vi "两边沿间隔_单点.vi"() -> ()   [LabVIEW 2013]
uses:
  <userlib>/ArtDAQ/_SubVI/ArtDAQ_CreateCITwoEdgeSepChan.vi
  <userlib>/ArtDAQ/_SubVI/ArtDAQ_Read Counter DBL 1Samp.vi
panel:
  out "H":dbl
  in  "第二个边沿":i32(ring)=10280 items=["上升"=10280, "下降"=10171]
  in  "第一个边沿":i32(ring)=10280 items=["上升"=10280, "下降"=10171]
  in  "Stop":bool
  in  "计数器":string="Dev1/ctr0"
  in  "最小值":dbl=1e-06 format="%0.6f"
  in  "MaxValue":dbl=10.0 caption="最大值" format="%0.6f"
  out "错误输出":errorcluster
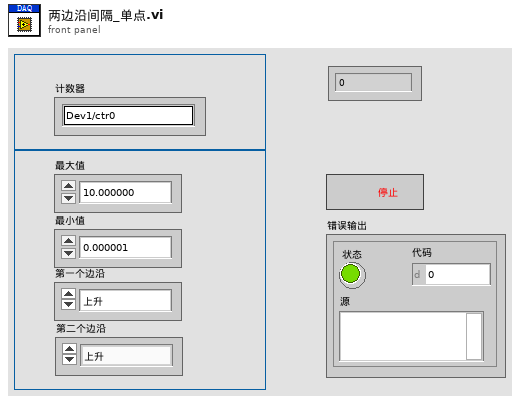
[diagram p1: front panel]
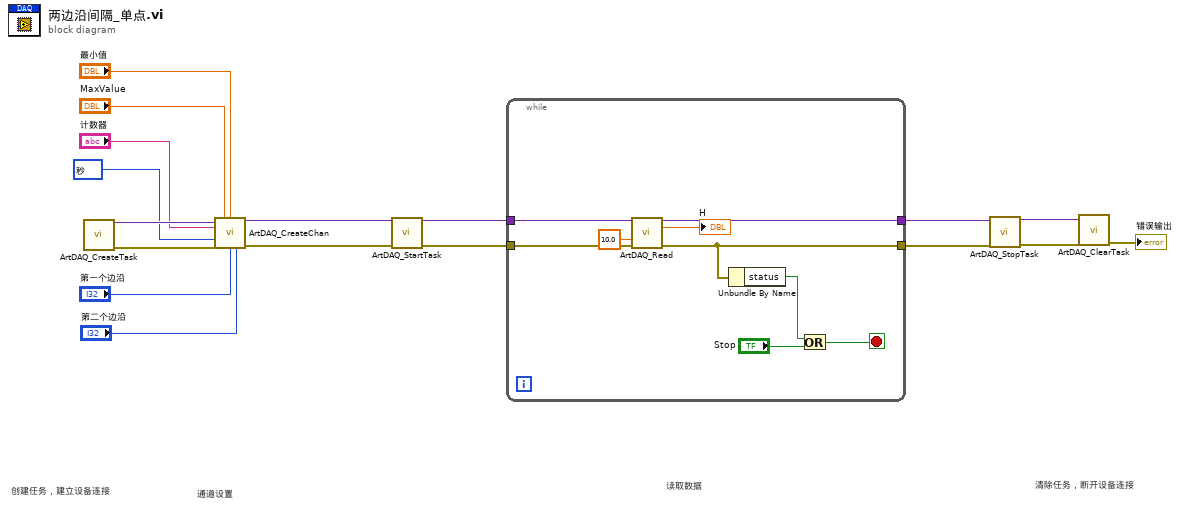
[diagram p0: block diagram]
diagram:
  w7 = 10364 items=["秒"=10364, "时钟滴答"=10304, "来自自定义换算"=10065] ("Units")
  # "清除任务，断开设备连接"
  # "读取数据"
  # "通道设置"
  # "创建任务，建立设备连接"
  n1 = call <userlib>:"ArtDAQ_CreateTask.vi"() -> ("任务句柄"=w17:variant, "错误输出"=w16:errorcluster)  [unwired: 14 in]
  n2 = call-poly <userlib>:"ArtDAQ_CreateChan.vi"("任务句柄"=w17, "最大值"="MaxValue", "最小值"="最小值", "计数器"="计数器", "单位"=w7, "错误输入"=w16, "第一个边沿"="第一个边沿", "第二个边沿"="第二个边沿") -> ("任务句柄"=w2:variant, "错误输出"=w1:errorcluster)  [unwired: 6 in]
  n3 = call <userlib>:"ArtDAQ_StartTask.vi"("任务句柄"=w2, "错误输入"=w1) -> ("任务句柄"=w4:variant, "错误输出"=w3:errorcluster)  [unwired: 12 in]
  n4 = while {
    tunnel: [w26] -> w14
    tunnel: [w25] -> w12
    tunnel: w4 -> [w24]
    tunnel: w3 -> [w23]
    stop <- w19 stop-if-true
    n5 = call-poly <userlib>:"ArtDAQ_Read.vi"("任务句柄"=w24, "超时s"=10.0 ("Timeout"), "错误输入"=w23) -> ("任务句柄"=w26:variant, "数据"=→"H":dbl, "错误输出"=w25:errorcluster)  [unwired: 10 in]
    n6 = Unbundle By Name(w25) -> ("status"=w21:bool)
    n7 = Or(x=w21, y="Stop") -> (x .or. y?=w19:bool)
  }
  n8 = call <userlib>:"ArtDAQ_StopTask.vi"("任务句柄"=w14, "错误输入"=w12) -> ("任务句柄"=w13:variant, "错误输出"=w11:errorcluster)  [unwired: 12 in]
  n9 = call <userlib>:"ArtDAQ_ClearTask.vi"("任务句柄"=w13, "错误输入"=w11) -> ("错误输出"=→"错误输出":errorcluster)  [unwired: 13 in]
